vi "spi_read_id.vi"(5 "COM":bool, 7 "VISA name":refnum<visa-resource-name>, 11 "data":u8[](array[numeric])) -> (3 "return":i32)   [LabVIEW 2016]
panel:
  in  "tVdCmdHeader":T1
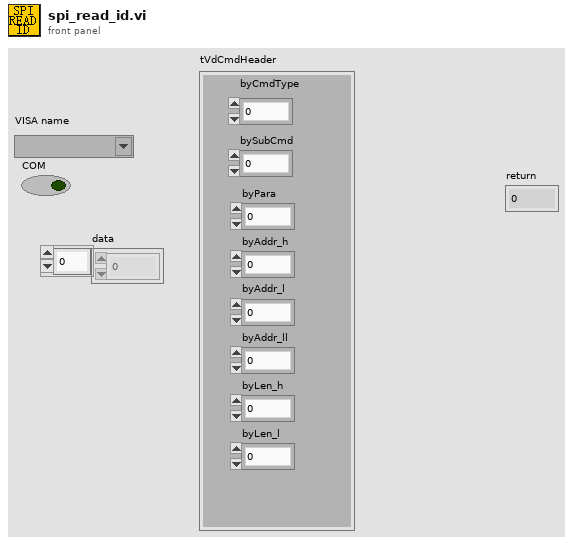
[diagram p1: front panel]
types:
  T1 = cluster{"byCmdType":u8, "bySubCmd":u8, "byPara":u8, "byAddr_h":u8, "byAddr_l":u8, "byAddr_ll":u8, "byLen_h ":u8, "byLen_l":u8}
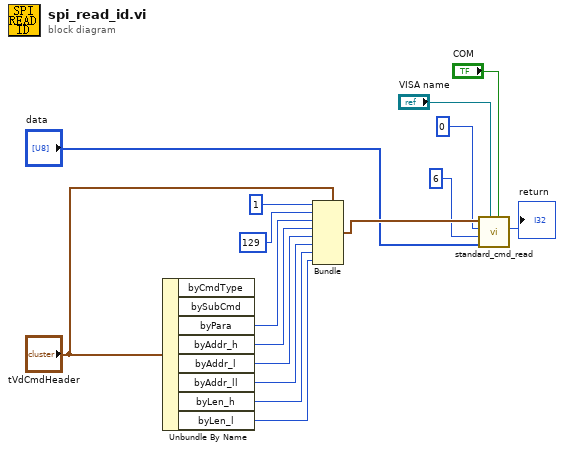
[diagram p0: block diagram]
diagram:
  n1 = Unbundle By Name("tVdCmdHeader") -> ("byPara"=w13:u8, "byAddr_h"=w12:u8, "byAddr_l"=w11:u8, "byAddr_ll"=w10:u8, "byLen_h"=w9:u8, "byLen_l"=w8:u8)  [unwired: 2 out]
  n2 = Bundle(cluster="tVdCmdHeader", "byCmdType"=u8 1, "bySubCmd"=u8 129, "byPara"=w13, "byAddr_h"=w12, "byAddr_l"=w11, "byAddr_ll"=w10, "byLen_h"=w9, "byLen_l"=w8) -> (w7:T1)
  n3 = call "standard_cmd_read.vi"("COM"="COM", "VISA name"="VISA name", "data"="data", "dwLen"=u32 6, "dwAddr"=u32 0, "cmd_std_header_t"=w7) -> ("return"=→"return":i32)  [unwired: 4 in, 1 out]
